vi "Number of Columns.vi"(8 "error in (no error)":errorcluster, 11 "PQ Result in":refnum<class "PQ Result.lvclass">) -> (0 "error out":errorcluster, 2 "Number of Columns":i32, 3 "PQ Result out":refnum<class "PQ Result.lvclass">)   [LabVIEW 2015, in "PQ Result.lvclass"]
uses:
  PQ Result.lvclass
  PQ Result.lvclass/PQ Result.ctl
  Connection/libpq.dll
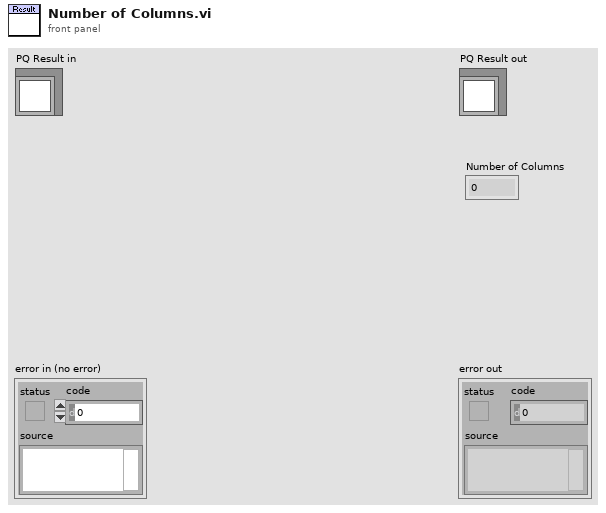
[diagram p1: front panel]
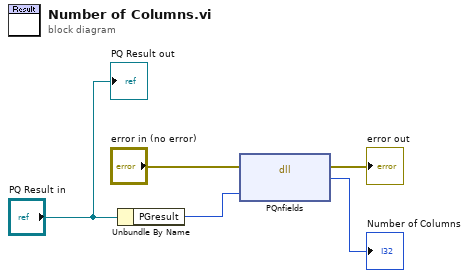
[diagram p0: block diagram]
diagram:
  n1 = Unbundle By Name("PQ Result in") -> ("PGresult"=w1:u32)
  n2 = dll-call lib="C:/PQ/Connection/libpq.dll" fn="PQnfields"(error in="error in (no error)", "PGresult"=w1) -> (error out=→"error out":errorcluster, "PQnfields"=→"Number of Columns":i32)  [unwired: 3 in, 1 out]
  "PQ Result out" <- "PQ Result in"
